vi "VM_ProjetoV5.1.vi"() -> ()   [LabVIEW 2016, in "Projeto_Modbus_Finalizado.lvlib"]
uses:
  Projeto_Modbus_Finalizado.lvlib
  <vilib>/userdefined/High Color/IMAQdx.ctl
  <vilib>/Analysis/baseanly.llb/Mean (DBL).vi
  <vilib>/lvdsc/process/Deploy Library.vi
  <vilib>/Utility/file.llb/Read Delimited Spreadsheet (DBL).vi
  <vilib>/Utility/file.llb/Write Delimited Spreadsheet (DBL).vi
  <vilib>/lvdsc/process/Undeploy Library.vi
  <vilib>/vision/driver/NI_Vision_Acquisition_Software.lvlib
  <resource>/objmgr/imaqdx.rc
  <vilib>/Analysis/NI_AALBase.lvlib
  <vilib>/lvdsc/NI_DSC.lvlib
panel:
  in  "Calibração\nRobô":path=path "C:/Users/rodrigorg1/Desktop/Projeto/calibracaoRobo.csv"
  in  "Calibração\nMesa":path=path "C:/Users/rodrigorg1/Desktop/Projeto/calibracaoMesa.csv"
  out "Error Out":errorcluster
  in  "Cut Limit":dbl=55.0 format="%#_13g"
  in  "Confirma":bool
  out "Status":string
  out "Câmera Robo":T1(plugin-control)
  out "Câmera Mesa":T1(plugin-control)
  in  "Começa jogada":bool
  in  "stop":bool
  in  "Source Câmera Robo":T2="S1156978"
  in  "Source Câmera Mesa":T2="cam0"
  out "Dobrao":bool
  out "Passa Vez":bool
  out "place pos Norm":dbl[](array[numeric])
  out "pick pos Norm":dbl[](array[numeric])
  out "place angle":dbl
  out "pick angle":dbl
  # "x 91\ny 176"
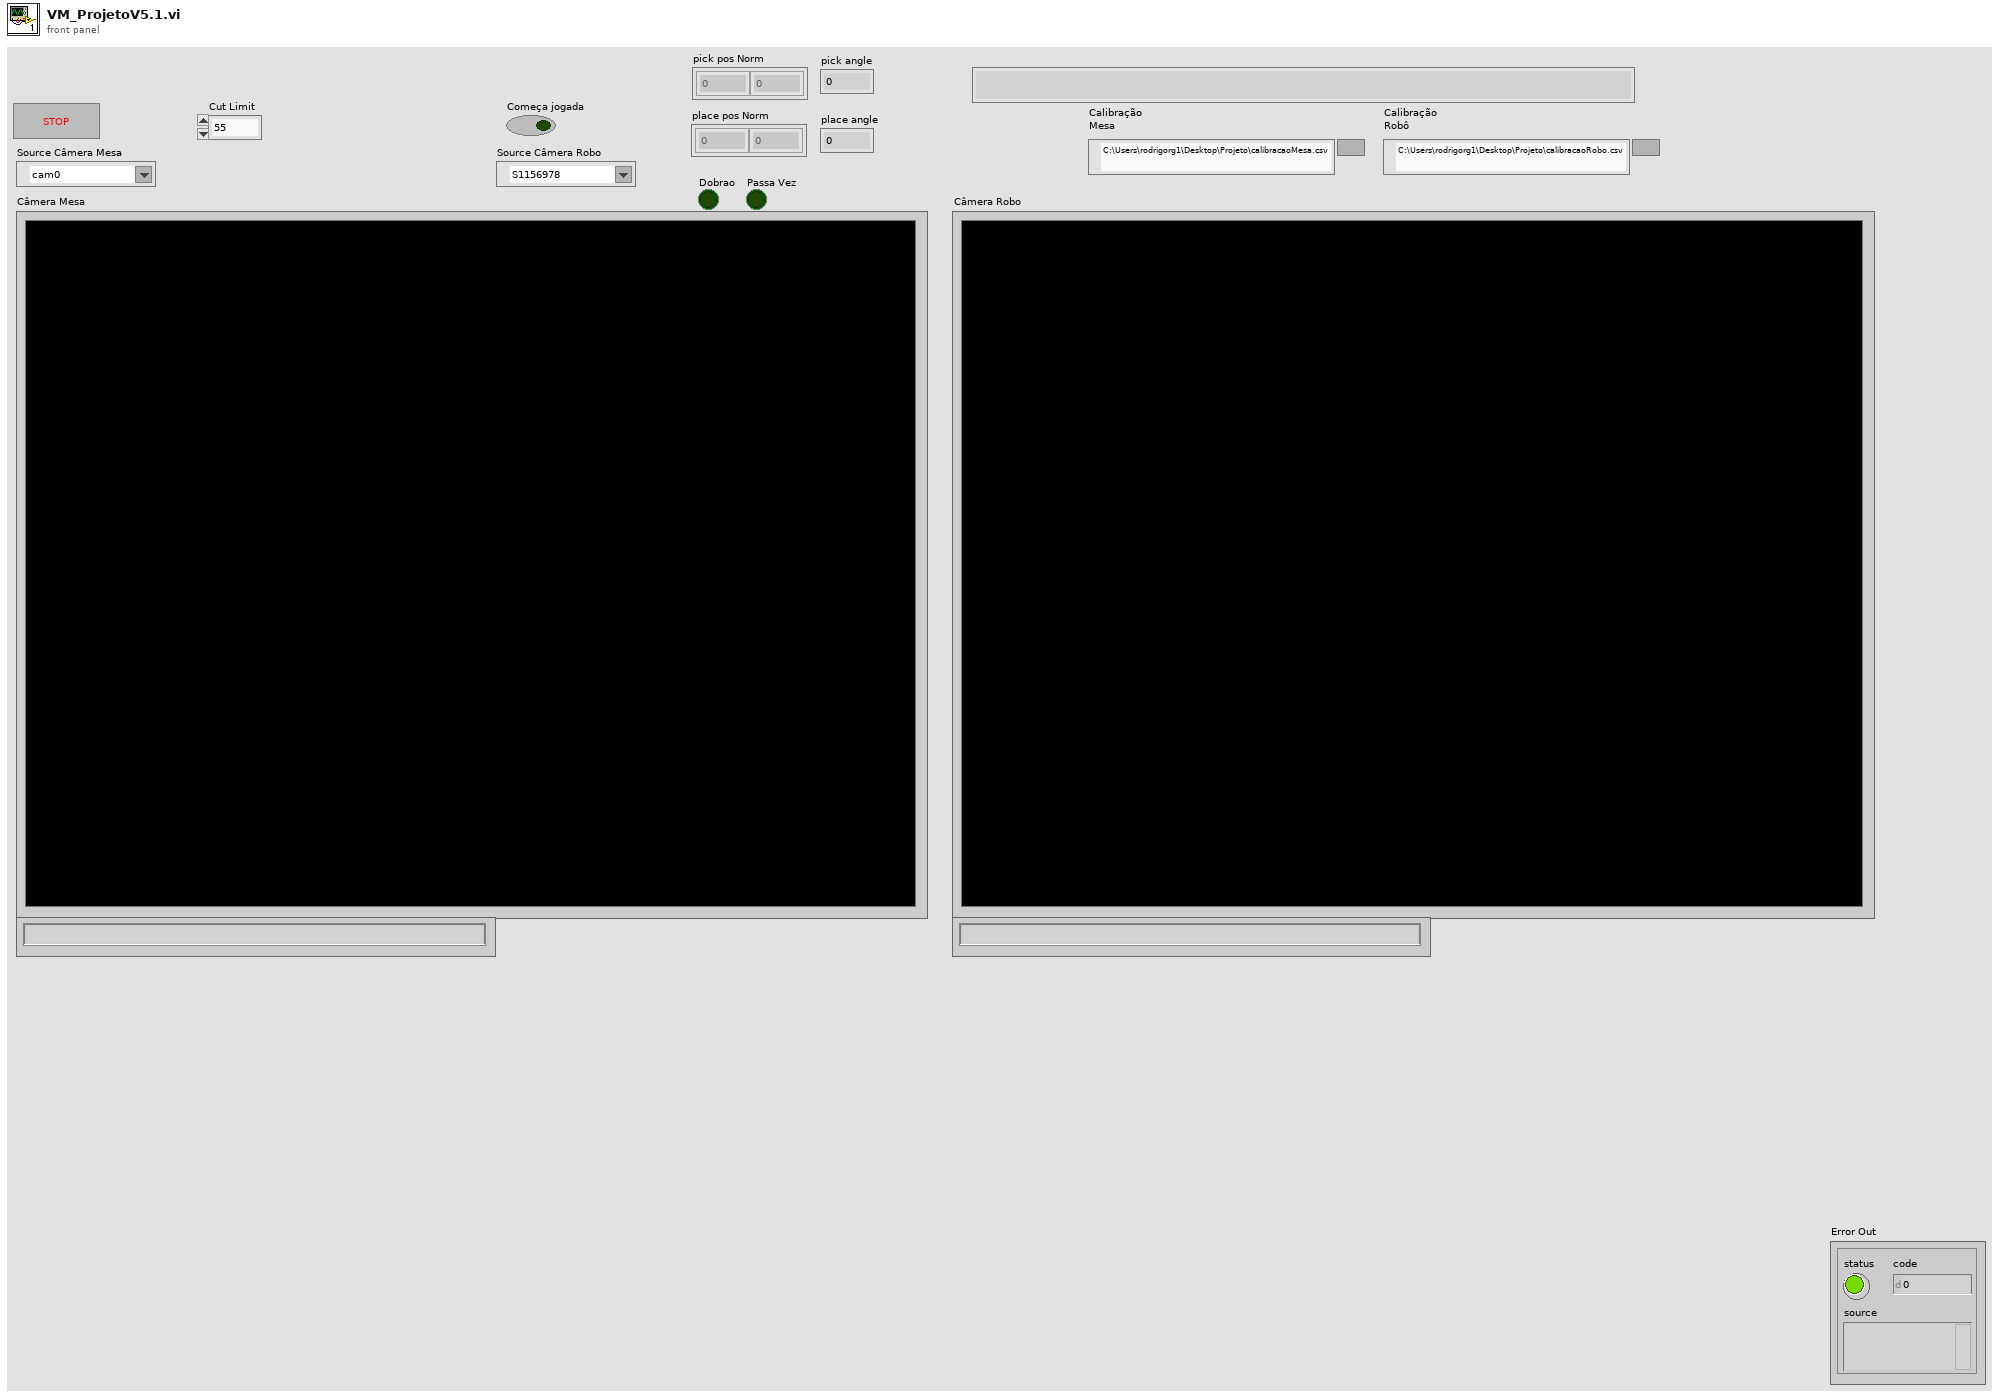
[diagram p1: front panel]
types:
  T1 = typedef "IMAQ Image.ctl" = refnum<image>
  T2 = typedef "IMAQdx.ctl" = refnum<k21>
  T3 = typedef "IMAQ Rectangle" = cluster{"Left":i32, "Top":i32, "Right":i32, "Bottom":i32, "Rotation":dbl}
  T4 = typedef "ROI Descriptor" = cluster{"Global Rectangle":i32[], "Contours":cluster{"ID":enum32{"External", "Internal"}, "Type":u32, "Coordinates":i32[]}[]}
  T5 = cluster{"Position":cluster{"x":sgl, "y":sgl}, "Angle":sgl, "Scale":sgl, "Score":sgl, "Bounding Box":cluster{"x":sgl, "y":sgl}[]}[]
  T6 = cluster{"Centro Peça":dbl[], "Centros Númeors":dbl[][], "Números":u8[], "ROI Números":T4[]}[]
  T7 = cluster{"Centro Peça":dbl[], "Centros Númeors":dbl[][], "Números":u8[], "ROI Números":T4[]}
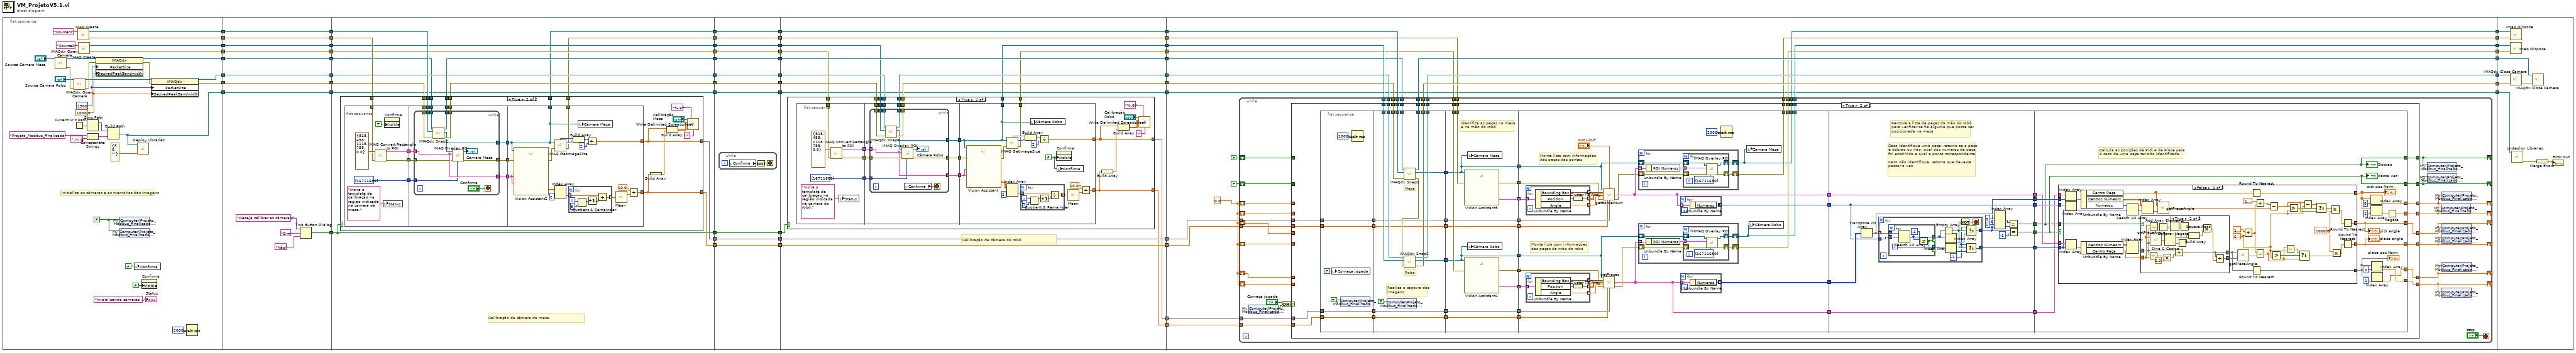
[diagram p0: block diagram]
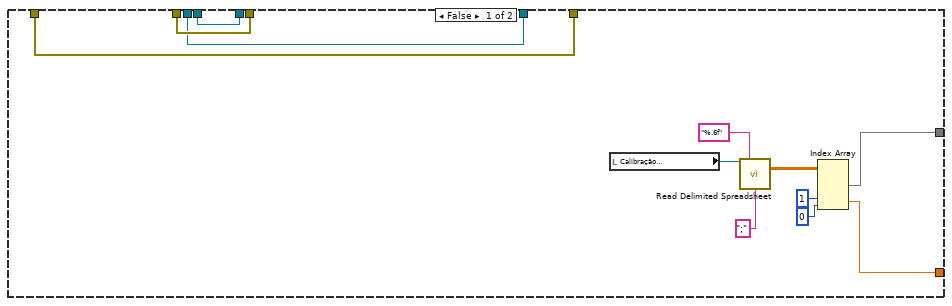
[diagram p2: hidden frame]
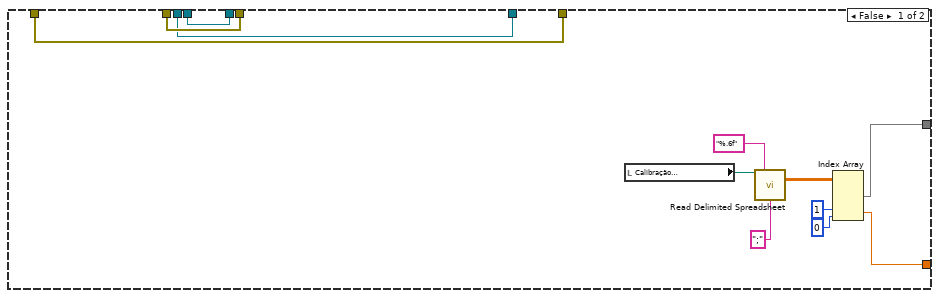
[diagram p3: hidden frame]
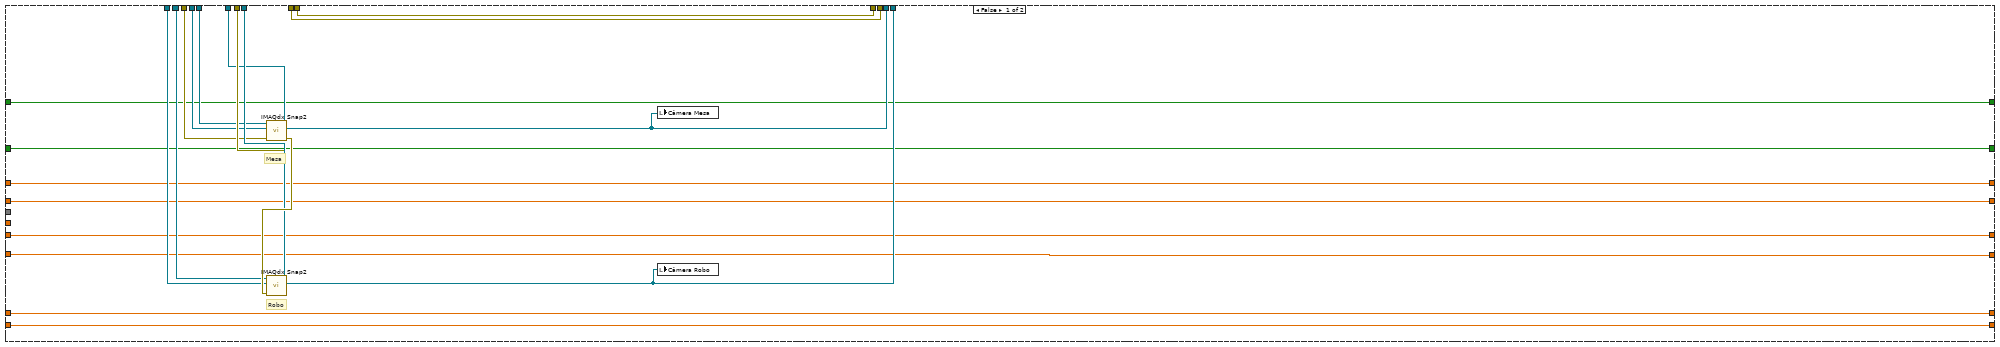
[diagram p4: hidden frame]
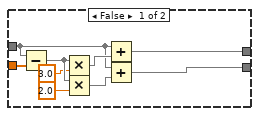
[diagram p5: hidden frame]
diagram:
  n1 = flat-sequence {
    tunnel: [w85] -> w17
    tunnel: [w84] -> w15
    tunnel: [w79] -> w13
    tunnel: [w83] -> w11
    tunnel: [w82] -> w9
    tunnel: [w78] -> w7
    tunnel: [w69] -> w5
    tunnel: [w61] -> w3
    tunnel: w17 -> [w101]
    tunnel: [w101] -> w16
    tunnel: w15 -> [w100]
    tunnel: [w100] -> w14
    tunnel: w13 -> [w99]
    tunnel: [w99] -> w12
    tunnel: w11 -> [w98]
    tunnel: [w98] -> w10
    tunnel: w9 -> [w97]
    tunnel: [w97] -> w8
    tunnel: w7 -> [w96]
    tunnel: [w96] -> w6
    tunnel: w5 -> [w95]
    tunnel: [w95] -> w4
    tunnel: w3 -> [w94]
    tunnel: [w94] -> w2
    tunnel: [w90] -> w1
    tunnel: w16 -> [w115]
    tunnel: w14 -> [w116]
    tunnel: w12 -> [w105]
    tunnel: w10 -> [w114]
    tunnel: w8 -> [w113]
    tunnel: w6 -> [w104]
    tunnel: [w109] -> w41
    tunnel: [w108] -> w39
    tunnel: [w114] -> w37
    tunnel: [w113] -> w35
    tunnel: [w112] -> w33
    tunnel: [w111] -> w31
    tunnel: w4 -> [w111]
    tunnel: [w110] -> w29
    tunnel: [w107] -> w27
    tunnel: [w106] -> w25
    tunnel: [w103] -> w20
    tunnel: w2 -> [w103]
    tunnel: [w102] -> w19
    tunnel: w1 -> [w102]
    tunnel: w41 -> [w213]
    tunnel: [w213] -> w40
    tunnel: w39 -> [w212]
    tunnel: [w212] -> w38
    tunnel: w37 -> [w211]
    tunnel: [w211] -> w36
    tunnel: w35 -> [w210]
    tunnel: [w210] -> w34
    tunnel: w33 -> [w209]
    tunnel: [w209] -> w32
    tunnel: w31 -> [w208]
    tunnel: [w208] -> w30
    tunnel: w29 -> [w207]
    tunnel: [w207] -> w28
    tunnel: w27 -> [w206]
    tunnel: [w206] -> w26
    tunnel: w25 -> [w205]
    tunnel: [w205] -> w24
    tunnel: [w204] -> w21
    tunnel: w20 -> [w204]
    tunnel: w19 -> [w203]
    tunnel: [w203] -> w18
    tunnel: w40 -> [w232]
    tunnel: [w232] -> w52
    tunnel: w38 -> [w231]
    tunnel: [w231] -> w51
    tunnel: w36 -> [w223]
    tunnel: [w222] -> w50
    tunnel: w34 -> [w221]
    tunnel: [w220] -> w49
    tunnel: w32 -> [w230]
    tunnel: [w230] -> w48
    tunnel: w30 -> [w225]
    tunnel: [w224] -> w47
    tunnel: w28 -> [w227]
    tunnel: [w226] -> w46
    tunnel: w26 -> [w229]
    tunnel: [w229] -> w45
    tunnel: w24 -> [w228]
    tunnel: [w228] -> w44
    tunnel: [w219] -> w43
    tunnel: [w218] -> w42
    tunnel: [w217] -> w22
    tunnel: w21 -> [w217]
    tunnel: w18 -> [w216]
    tunnel: [w337] -> w59
    tunnel: [w340] -> w58
    tunnel: [w334] -> w57
    tunnel: [w339] -> w56
    tunnel: [w338] -> w55
    tunnel: [w336] -> w54
    tunnel: [w335] -> w53
    tunnel: w52 -> [w333]
    tunnel: w51 -> [w332]
    tunnel: w50 -> [w331]
    tunnel: w49 -> [w330]
    tunnel: w48 -> [w329]
    tunnel: w47 -> [w328]
    tunnel: w46 -> [w327]
    tunnel: w45 -> [w325]
    tunnel: w44 -> [w326]
    tunnel: w43 -> [w323]
    tunnel: w42 -> [w324]
    tunnel: [w322] -> w23
    tunnel: w22 -> [w322]
    tunnel: w59 -> [w681]
    tunnel: w58 -> [w679]
    tunnel: w57 -> [w683]
    tunnel: w56 -> [w686]
    tunnel: w55 -> [w685]
    tunnel: w54 -> [w682]
    tunnel: w53 -> [w684]
    tunnel: w23 -> [w676]
    frame #0 {
      w60 = FALSE ("000021")
      w73 = 1000.0 ("DesiredPeakBandwidth")
      w74 = u32 1500 ("PacketSize")
      # "Inicializa as câmeras e as memórias das imagens"
      n2 = call <vilib>:"IMAQdx Open Camera.vi"("Session In"="Source Câmera Mesa") -> ("error out"=w77:errorcluster, "Session Out"=w80:T2)  [unwired: 9 in]
      n3 = Current VI's Path() -> (path=w62:path)
      n4 = call <vilib>:"IMAQdx Open Camera.vi"("error in"=w77, "Session In"="Source Câmera Robo") -> ("error out"=w76:errorcluster, "Session Out"=w81:T2)  [unwired: 8 in]
      n5 = call "IMAQ Create"("Image Name"="SourceM") -> ("New Image"=w85:T1, "error out"=w84:errorcluster)  [unwired: 4 in]
      n6 = call "IMAQ Create"("Image Name"="SourceR") -> ("New Image"=w83:T1, "error out"=w82:errorcluster)  [unwired: 4 in]
      n7 = Strip Path(path=w62) -> (stripped path=w63:path)  [unwired: 1 out]
      n8 = Concatenate Strings("Projeto_Modbus_Finalizado" ("library path"), ".lvlib" ("string")) -> (w66:string)
      n9 = property class="IMAQdx"(reference=w80, error in=w76, "PacketSize"=w74, "DesiredPeakBandwidth"=w73) -> (reference out=w79:T2, error out=w75:errorcluster)
      n10 = Build Path(base path=w63, name or relative path=w66) -> (appended path=w61:path)
      n11 = shared-variable "My Computer\\Projeto_Modbus_Finalizado.lvlib\\000021"(w60) -> ()  [unwired: 1 in, 1 out]
      n12 = shared-variable "My Computer\\Projeto_Modbus_Finalizado.lvlib\\000020"(w60) -> ()  [unwired: 1 in, 1 out]
      n13 = local write "Confirma"(FALSE ("Confirma")) -> ()
      n14 = call-poly <vilib>:"Deploy Libraries.vi"("error in (no error)"=errorcluster {"status"=FALSE, "code"=0, "source"=""}, "library path"=w61) -> ()  [unwired: 7 in, 1 out]
      n15 = property on="Confirma" class="Bool (strict)"("Visible"=FALSE) -> ()  [unwired: 2 in, 2 out]
      n16 = property class="IMAQdx"(reference=w81, error in=w75, "PacketSize"=w74, "DesiredPeakBandwidth"=w73) -> (reference out=w69:T2, error out=w78:errorcluster)
      n17 = Wait (ms)(milliseconds to wait=u32 2000) -> ()  [unwired: 1 out]
      "Status" <- "Inicializando câmeras ..." ("Status")
    }
    frame #1 {
      n18 = Two Button Dialog(message="Deseja calibrar as câmeras?", 1:"Não" ("F button name (\"Cancel\")"), 2:"Sim" ("T button name (\"OK\")")) -> (T button?=w90:bool)
    }
    frame #2 {
      # "Calibração da câmera da mesa"
      n19 = case shown="True" w102 {
        tunnel: w116 -> [w125 w143]
        tunnel: w115 -> [w126 w142]
        tunnel: [w127 w141] -> w112
        tunnel: [w128 w140] -> w110
        tunnel: [w126 w139] -> w109
        tunnel: [w125 w138] -> w108
        tunnel: [w118 w133] -> w107
        tunnel: [w117 w134] -> w106
        tunnel: w105 -> [w127 w137]
        tunnel: w104 -> [w128 w136]
        frame False {
          n20 = local read "Calibração\nMesa"() -> (w124:path)
          n21 = call-poly <vilib>:"Read Delimited Spreadsheet.vi"("file path (dialog if empty)"=w124, "format (%.3f)"="%.6f", "delimiter (\\t)"=";" ("delimiter (\\t)")) -> ("all rows"=w121:dbl[][])  [unwired: 7 in, 5 out]
          n22 = Index Array(array=w121, index (row) #2=1, index (col) #2=0) -> (element #1=w117:dbl[], element #2=w118:dbl)  [unwired: 2 in]
        }
        frame True {
          n23 = flat-sequence {
            tunnel: w143 -> [w154]
            tunnel: [w152] -> w149
            tunnel: [w151] -> w148
            tunnel: [u32[] [16711680] ("Colors (Green)")] -> w147
            tunnel: w137 -> [w167]
            tunnel: w136 -> [w166]
            tunnel: w142 -> [w165]
            tunnel: [w164] -> w141
            tunnel: [w163] -> w140
            tunnel: w149 -> [w162]
            tunnel: w148 -> [w161]
            tunnel: [w160] -> w146
            tunnel: [w159] -> w145
            tunnel: [w158] -> w144
            tunnel: w147 -> [w157]
            tunnel: w146 -> [w196]
            tunnel: w145 -> [w195]
            tunnel: [w187] -> w133
            tunnel: w144 -> [w180]
            tunnel: [w180] -> w139
            tunnel: [w182] -> w138
            tunnel: [w181] -> w134
            frame #0 {
              n24 = call "IMAQ Convert Rectangle to ROI"("error in (no error)"=w154, "Rectangle"=T3 {"Left"=818, "Top"=458, "Right"=1118, "Bottom"=758, "Rotation"=0.0}) -> ("error out"=w152:errorcluster, "ROI Descriptor"=w151:T4)  [unwired: 7 in]
              n25 = local write "Status"("Insira o template de calibração na região indicada na câmera da mesa." ("Status")) -> ()
              n26 = property on="Confirma" class="Bool (strict)"("Visible"=TRUE) -> ()  [unwired: 2 in, 2 out]
            }
            frame #1 {
              n27 = while {
                tunnel: w167 -> [w178]
                tunnel: w166 -> [w177]
                tunnel: w165 -> [w176]
                tunnel: [w175] -> w164
                tunnel: [w174] -> w163
                tunnel: w162 -> [w168]
                tunnel: w161 -> [w171]
                tunnel: [w173] -> w160
                tunnel: [w171] -> w159
                tunnel: [w169] -> w158
                tunnel: w157 -> [w170]
                stop <- "Confirma" stop-if-true
                n28 = call <vilib>:"IMAQdx Snap2.vi"("error in"=w177, "Image In"=w176, "Session In"=w178) -> ("error out"=w174:errorcluster, "Image Out"=w169:T1, "Session Out"=w175:T2)  [unwired: 6 in]
                n29 = call "IMAQ Overlay ROI"("Colors (Green)"=w170, "error in (no error)"=w168, "ROI Descriptor"=w171, "Image"=w169) -> ("error out"=w173:errorcluster, "Image Out"=→"Câmera Mesa":T1)  [unwired: 6 in]
              }
            }
            frame #2 {
              n30 = call "Vision Assistant2"("Image In"=w180, "ROI Descriptor (Adv. Straight Edge 1)"=w195, "ROI Descriptor (Copy of Adv. Straight Edge 1)"=w195, "error in"=w196) -> ("Caliper Results (Caliper 2)"=w194:sgl[][], "error out"=w188:errorcluster)  [unwired: 21 in, 1 out]
              n31 = call "IMAQ GetImageSize"("Image"=w180, "error in (no error)"=w188) -> ("Y Resolution"=w186:i32, "X Resolution"=w185:i32, "error out"=w182:errorcluster)  [unwired: 2 in]
              n32 = Index Array(array=w194, index (col)=2 ("disabled index (col)")) -> (element=w192:sgl[])  [unwired: 1 in]
              n33 = for {
                tunnel: w192 -> [w199] mode=indexing
                tunnel: [w197] -> w191 mode=indexing
                i -> [w202]
                n34 = Quotient & Remainder(x=w202, y=5) -> (x-y*floor(x/y)=w200:i32)  [unwired: 1 out]
                n35 = Increment(x=w200) -> (x+1=w198:i32)
                n36 = Divide(x=w199, y=w198) -> (x/y=w197:sgl)
              }
              n37 = Build Array(w185, w186) -> (w184:i32[])
              n38 = local write "Câmera Mesa"(w180) -> ()
              n39 = Divide(x=w184, y=2) -> (x/y=w181:dbl[])
              n40 = call-poly <vilib>:"Mean.vi"("X"=w191) -> ("mean"=w190:dbl)  [unwired: 1 out]
              n41 = Divide(x=10.0, y=w190) -> (x/y=w187:dbl)
            }
          }
          n42 = Build Array(w133) -> (w132:dbl[])
          n43 = Build Array(w134, w132) -> (w131:dbl[][])
          n44 = call-poly <vilib>:"Write Delimited Spreadsheet.vi"("file path (dialog if empty)"="Calibração\nMesa", "format (%.3f)"="%.6f", "2D data"=w131, "delimiter (\\t)"=";" ("delimiter (\\t)")) -> ()  [unwired: 10 in, 2 out]
        }
      }
    }
    frame #3 {
      n45 = while {
        stop <- w215 stop-if-true
        n46 = local read "Confirma"() -> (w214:bool)
        n47 = Not(x=w214) -> (.not. x?=w215:bool)
      }
    }
    frame #4 {
      # "Calibração da câmera do robô"
      n48 = case shown="True" w216 {
        tunnel: w227 -> [w243 w259]
        tunnel: [w243 w258] -> w226
        tunnel: w225 -> [w244 w257]
        tunnel: [w244 w256] -> w224
        tunnel: w223 -> [w242 w255]
        tunnel: [w242 w254] -> w222
        tunnel: w221 -> [w241 w253]
        tunnel: [w241 w252] -> w220
        tunnel: [w233 w246] -> w219
        tunnel: [w234 w245] -> w218
        frame False {
          n49 = local read "Calibração\nRobô"() -> (w235:path)
          n50 = call-poly <vilib>:"Read Delimited Spreadsheet.vi"("file path (dialog if empty)"=w235, "format (%.3f)"="%.6f", "delimiter (\\t)"=";" ("delimiter (\\t)")) -> ("all rows"=w238:dbl[][])  [unwired: 7 in, 5 out]
          n51 = Index Array(array=w238, index (row) #2=1, index (col) #2=0) -> (element #1=w234:dbl[], element #2=w233:dbl)  [unwired: 2 in]
        }
        frame True {
          n52 = flat-sequence {
            tunnel: w253 -> [w270]
            tunnel: [w269] -> w265
            tunnel: [w268] -> w264
            tunnel: [u32[] [16711680] ("Colors (Green)")] -> w263
            tunnel: w257 -> [w282]
            tunnel: w259 -> [w281]
            tunnel: w255 -> [w280]
            tunnel: [w279] -> w256
            tunnel: [w278] -> w258
            tunnel: w265 -> [w277]
            tunnel: w264 -> [w276]
            tunnel: [w275] -> w262
            tunnel: [w274] -> w261
            tunnel: [w273] -> w260
            tunnel: w263 -> [w272]
            tunnel: w262 -> [w312]
            tunnel: w261 -> [w311]
            tunnel: [w303] -> w246
            tunnel: w260 -> [w296]
            tunnel: [w296] -> w254
            tunnel: [w298] -> w252
            tunnel: [w297] -> w245
            frame #0 {
              n53 = call "IMAQ Convert Rectangle to ROI"("error in (no error)"=w270, "Rectangle"=T3 {"Left"=818, "Top"=458, "Right"=1118, "Bottom"=758, "Rotation"=0.0}) -> ("error out"=w269:errorcluster, "ROI Descriptor"=w268:T4)  [unwired: 7 in]
              n54 = local write "Status"("Insira o template de calibração na região indicada na câmera do robô." ("Status")) -> ()
            }
            frame #1 {
              n55 = while {
                tunnel: w282 -> [w294]
                tunnel: w281 -> [w293]
                tunnel: w280 -> [w292]
                tunnel: [w291] -> w279
                tunnel: [w290] -> w278
                tunnel: w277 -> [w289]
                tunnel: w276 -> [w287]
                tunnel: [w288] -> w275
                tunnel: [w287] -> w274
                tunnel: [w286] -> w273
                tunnel: w272 -> [w285]
                stop <- w283 stop-if-true
                n56 = call <vilib>:"IMAQdx Snap2.vi"("error in"=w293, "Image In"=w292, "Session In"=w294) -> ("error out"=w290:errorcluster, "Image Out"=w286:T1, "Session Out"=w291:T2)  [unwired: 6 in]
                n57 = call "IMAQ Overlay ROI"("Colors (Green)"=w285, "error in (no error)"=w289, "ROI Descriptor"=w287, "Image"=w286) -> ("error out"=w288:errorcluster, "Image Out"=→"Câmera Robo":T1)  [unwired: 6 in]
                n58 = local read "Confirma"() -> (w283:bool)
              }
            }
            frame #2 {
              w295 = FALSE ("Visible")
              n59 = call "Vision Assistant"("Image In"=w296, "ROI Descriptor (Adv. Straight Edge 1)"=w311, "ROI Descriptor (Copy of Adv. Straight Edge 1)"=w311, "error in"=w312) -> ("Caliper Results (Caliper 2)"=w310:sgl[][], "error out"=w304:errorcluster)  [unwired: 21 in, 1 out]
              n60 = call "IMAQ GetImageSize"("Image"=w296, "error in (no error)"=w304) -> ("Y Resolution"=w302:i32, "X Resolution"=w301:i32, "error out"=w298:errorcluster)  [unwired: 2 in]
              n61 = Index Array(array=w310, index (col)=2 ("disabled index (col)")) -> (element=w308:sgl[])  [unwired: 1 in]
              n62 = for {
                tunnel: w308 -> [w315] mode=indexing
                tunnel: [w313] -> w307 mode=indexing
                i -> [w318]
                n63 = Quotient & Remainder(x=w318, y=5) -> (x-y*floor(x/y)=w316:i32)  [unwired: 1 out]
                n64 = Increment(x=w316) -> (x+1=w314:i32)
                n65 = Divide(x=w315, y=w314) -> (x/y=w313:sgl)
              }
              n66 = Build Array(w301, w302) -> (w300:i32[])
              n67 = local write "Câmera Robo"(w296) -> ()
              n68 = Divide(x=w300, y=2) -> (x/y=w297:dbl[])
              n69 = property on="Confirma" class="Bool (strict)"("Visible"=w295) -> ()  [unwired: 2 in, 2 out]
              n70 = local write "Confirma"(w295) -> ()
              n71 = call-poly <vilib>:"Mean.vi"("X"=w307) -> ("mean"=w306:dbl)  [unwired: 1 out]
              n72 = Divide(x=10.0, y=w306) -> (x/y=w303:dbl)
            }
          }
          n73 = Build Array(w246) -> (w250:dbl[])
          n74 = Build Array(w245, w250) -> (w249:dbl[][])
          n75 = call-poly <vilib>:"Write Delimited Spreadsheet.vi"("file path (dialog if empty)"="Calibração\nRobô", "format (%.3f)"="%.6f", "2D data"=w249, "delimiter (\\t)"=";" ("delimiter (\\t)")) -> ()  [unwired: 10 in, 2 out]
        }
      }
    }
    frame #5 {
      w319 = 0.0 ("Numeric")
      n76 = while {
        tunnel: w329 -> [w378]
        tunnel: w333 -> [w377]
        tunnel: w331 -> [w376]
        tunnel: w328 -> [w375]
        tunnel: w327 -> [w374]
        tunnel: [w373] -> w340
        tunnel: [w372] -> w339
        tunnel: [w371] -> w338
        tunnel: w332 -> [w370]
        tunnel: w330 -> [w369]
        tunnel: [w368] -> w337
        tunnel: [w367] -> w334
        tunnel: [w365] -> w336
        tunnel: [w364] -> w335
        tunnel: w326 -> [w363]
        tunnel: w325 -> [w362]
        tunnel: w324 -> [w361]
        tunnel: w323 -> [w360]
        shift-right: [w356] -> _
        shift-left: FALSE -> [w347]
        shift-right: [w355] -> _
        shift-left: FALSE -> [w348]
        shift-right: [w354] -> _
        shift-left: w319 -> [w346]
        shift-right: [w353] -> _
        shift-left: w319 -> [w345]
        shift-right: [w352] -> _
        shift-left: w319 -> [w344]
        shift-right: [w351] -> _
        shift-left: w319 -> [w343]
        shift-right: [w350] -> _
        shift-left: w319 -> [w342]
        shift-right: [w349] -> _
        shift-left: w319 -> [w341]
        stop <- "stop" stop-if-true
        n77 = shared-variable "My Computer\\Projeto_Modbus_Finalizado.lvlib\\000022"() -> (w357:bool)  [unwired: 1 in, 1 out]
        n78 = Or(x="Começa jogada", y=w357) -> (x .or. y?=w359:bool)
        n79 = case shown="True" w359 {
          tunnel: w378 -> [w390 w456]
          tunnel: w377 -> [w389 w455]
          tunnel: w376 -> [w396 w454]
          tunnel: w375 -> [w395 w453]
          tunnel: w374 -> [w392 w452]
          tunnel: [w391 w451] -> w373
          tunnel: [w394 w450] -> w372
          tunnel: [w393 w449] -> w371
          tunnel: w370 -> [w399 w447]
          tunnel: w369 -> [w398 w445]
          tunnel: [w388 w413] -> w368
          tunnel: [w387 w414] -> w367
          tunnel: [w399 w411] -> w365
          tunnel: [w398 w412] -> w364
          tunnel: w363 -> [_ w400]
          tunnel: w362 -> [_ w427]
          tunnel: w361 -> [_ w402]
          tunnel: w360 -> [_ w401]
          tunnel: [w384 w410] -> w354
          tunnel: [w382 w409] -> w353
          tunnel: [w383 w408] -> w352
          tunnel: [w381 w407] -> w351
          tunnel: [w380 w406] -> w350
          tunnel: [w379 w405] -> w349
          tunnel: [w385 w404] -> w356
          tunnel: [w386 w403] -> w355
          tunnel: w348 -> [w386 _]
          tunnel: w347 -> [w385 _]
          tunnel: w346 -> [w384 _]
          tunnel: w345 -> [w382 _]
          tunnel: w344 -> [w383 _]
          tunnel: w343 -> [w381 _]
          tunnel: w342 -> [w380 _]
          tunnel: w341 -> [w379 _]
          frame False {
            # "Robo"
            # "Mesa"
            n80 = call <vilib>:"IMAQdx Snap2.vi"("error in"=w392, "Image In"=w389, "Session In"=w390) -> ("error out"=w397:errorcluster, "Image Out"=w388:T1, "Session Out"=w391:T2)  [unwired: 6 in]
            n81 = call <vilib>:"IMAQdx Snap2.vi"("error in"=w397, "Image In"=w396, "Session In"=w395) -> ("error out"=w393:errorcluster, "Image Out"=w387:T1, "Session Out"=w394:T2)  [unwired: 6 in]
            n82 = local write "Câmera Mesa"(w388) -> ()
            n83 = local write "Câmera Robo"(w387) -> ()
          }
          frame True {
            n84 = flat-sequence {
              tunnel: w401 -> [w460]
              tunnel: w402 -> [w461]
              tunnel: w427 -> [w462]
              tunnel: w400 -> [w463]
              tunnel: [w463] -> w418
              tunnel: [w462] -> w417
              tunnel: [w461] -> w416
              tunnel: [w460] -> w415
              tunnel: w456 -> [w479]
              tunnel: w455 -> [w478]
              tunnel: w454 -> [w477]
              tunnel: w453 -> [w476]
              tunnel: w452 -> [w470]
              tunnel: [w475] -> w451
              tunnel: [w474] -> w450
              tunnel: [w473] -> w449
              tunnel: [w472] -> w448
              tunnel: [w471] -> w446
              tunnel: [w468] -> w425
              tunnel: [w467] -> w423
              tunnel: [w466] -> w421
              tunnel: [w465] -> w420
              tunnel: w418 -> [w468]
              tunnel: w417 -> [w467]
              tunnel: w416 -> [w466]
              tunnel: w415 -> [w465]
              tunnel: w448 -> [w481]
              tunnel: w447 -> [w491]
              tunnel: w446 -> [w480]
              tunnel: w445 -> [w490]
              tunnel: [w489] -> w444
              tunnel: [w488] -> w443
              tunnel: [w480] -> w442
              tunnel: [w481] -> w441
              tunnel: [w487] -> w440
              tunnel: [w486] -> w439
              tunnel: [w485] -> w426
              tunnel: w425 -> [w485]
              tunnel: [w484] -> w424
              tunnel: w423 -> [w484]
              tunnel: [w483] -> w422
              tunnel: w421 -> [w483]
              tunnel: w420 -> [w482]
              tunnel: [w482] -> w419
              tunnel: w444 -> [w519]
              tunnel: w443 -> [w518]
              tunnel: w442 -> [w493]
              tunnel: w441 -> [w494]
              tunnel: w440 -> [w514]
              tunnel: w439 -> [w510]
              tunnel: [w509] -> w438
              tunnel: [w508] -> w437
              tunnel: [w502] -> w436
              tunnel: [w500] -> w435
              tunnel: w426 -> [w507]
              tunnel: w424 -> [w506]
              tunnel: w422 -> [w505]
              tunnel: w419 -> [w504]
              tunnel: [w495] -> w414
              tunnel: [w498] -> w412
              tunnel: [w496] -> w413
              tunnel: [w497] -> w411
              tunnel: w438 -> [w558]
              tunnel: w437 -> [w565]
              tunnel: w436 -> [w564]
              tunnel: w435 -> [w560]
              tunnel: [w564] -> w434
              tunnel: [w563] -> w433
              tunnel: [w562] -> w432
              tunnel: [w561] -> w431
              tunnel: [w560] -> w430
              tunnel: [w559] -> w429
              tunnel: [w558] -> w428
              tunnel: w434 -> [w605]
              tunnel: w433 -> [w595]
              tunnel: w432 -> [w596]
              tunnel: w431 -> [w608]
              tunnel: w430 -> [w604]
              tunnel: w429 -> [w607]
              tunnel: w428 -> [w606]
              tunnel: [w597] -> w410
              tunnel: [w589] -> w409
              tunnel: [w594] -> w408
              tunnel: [w593] -> w407
              tunnel: [w591] -> w406
              tunnel: [w592] -> w405
              tunnel: [w596] -> w404
              tunnel: [w595] -> w403
              frame #0 {
                n85 = local write "Começa jogada"(FALSE ("Começa jogada")) -> ()
                n86 = shared-variable "My Computer\\Projeto_Modbus_Finalizado.lvlib\\000021"(TRUE ("000021")) -> ()  [unwired: 1 in, 1 out]
                n87 = Wait (ms)(milliseconds to wait=u32 1000) -> ()  [unwired: 1 out]
              }
              frame #1 {
                # "Realiza a captura das\nimagens"
                # "Robo"
                # "Mesa"
                n88 = shared-variable "My Computer\\Projeto_Modbus_Finalizado.lvlib\\000021"(FALSE ("000021")) -> ()  [unwired: 1 in, 1 out]
                n89 = call <vilib>:"IMAQdx Snap2.vi"("error in"=w470, "Image In"=w478, "Session In"=w479) -> ("error out"=w469:errorcluster, "Image Out"=w472:T1, "Session Out"=w475:T2)  [unwired: 6 in]
                n90 = call <vilib>:"IMAQdx Snap2.vi"("error in"=w469, "Image In"=w477, "Session In"=w476) -> ("error out"=w473:errorcluster, "Image Out"=w471:T1, "Session Out"=w474:T2)  [unwired: 6 in]
              }
              frame #2 {
                # "Identifica as peças na mesa\ne na mão do robô"
                n91 = call "Vision Assistant3"("Image In"=w481, "error in"=w491) -> ("Matches (Pattern Matching 1)"=w488:T5, "error out"=w487:errorcluster)  [unwired: 23 in, 1 out]
                n92 = call "Vision Assistant4"("Image In"=w480, "error in"=w490) -> ("Matches (Pattern Matching 1)"=w489:T5, "error out"=w486:errorcluster)  [unwired: 23 in, 1 out]
                n93 = local write "Câmera Mesa"(w481) -> ()
                n94 = local write "Câmera Robo"(w480) -> ()
              }
              frame #3 {
                # "Monta lista com informações\ndas peças das pontas"
                # "Monta lista com informações\ndas peças da mão do robô"
                n95 = for {
                  tunnel: w518 -> [w552] mode=indexing
                  tunnel: [w550] -> w516 mode=indexing
                  tunnel: [w549] -> w517 mode=indexing
                  tunnel: [w548] -> w515 mode=indexing
                  n96 = Unbundle By Name(w552) -> ("Bounding Box"=w549:cluster{"x":sgl, "y":sgl}[], "Position"=w551:cluster{"x":sgl, "y":sgl}, "Angle"=w548:sgl)
                  n97 = Cluster To Array(cluster=w551) -> (array=w550:sgl[])
                }
                n98 = for {
                  tunnel: w519 -> [w557] mode=indexing
                  tunnel: [w555] -> w512 mode=indexing
                  tunnel: [w554] -> w513 mode=indexing
                  tunnel: [w553] -> w511 mode=indexing
                  n99 = Unbundle By Name(w557) -> ("Bounding Box"=w554:cluster{"x":sgl, "y":sgl}[], "Position"=w556:cluster{"x":sgl, "y":sgl}, "Angle"=w553:sgl)
                  n100 = Cluster To Array(cluster=w556) -> (array=w555:sgl[])
                }
                n101 = call "getBorderNum.vi"("Refnum in"=w494, "Cut Limit"="Cut Limit", "Bounding Box"=w517, "Position"=w516, "Angle"=w515, "error in (no error)"=w514, "Step"=w506, "Origin Pixel"=w507) -> ("Data Pieces"=w502:T6, "error out"=w501:errorcluster)  [unwired: 5 in, 1 out]
                n102 = call "getPieces.vi"("Refnum in"=w493, "Bounding Box"=w513, "Position"=w512, "Angle"=w511, "error in (no error)"=w510, "Step"=w504, "Origin Pixel"=w505) -> ("Data Pieces"=w500:T6, "error out"=w499:errorcluster)  [unwired: 6 in, 1 out]
                n103 = for {
                  tunnel: w502 -> [w537] mode=indexing
                  shift-right: [w534] -> w496
                  shift-left: w494 -> [w535]
                  shift-right: [w532] -> w497
                  shift-left: w501 -> [w533]
                  n104 = Unbundle By Name(w537) -> ("ROI Números"=w536:T4[])
                  n105 = for {
                    tunnel: w536 -> [w543] mode=indexing
                    shift-right: [w541] -> w534
                    shift-left: w535 -> [w542]
                    shift-right: [w539] -> w532
                    shift-left: w533 -> [w540]
                    n106 = call "IMAQ Overlay ROI"("Colors (Green)"=u32[] [16711680], "error in (no error)"=w540, "ROI Descriptor"=w543, "Image"=w542) -> ("error out"=w539:errorcluster, "Image Out"=w541:T1)  [unwired: 6 in]
                  }
                }
                n107 = for {
                  tunnel: w500 -> [w525] mode=indexing
                  shift-right: [w522] -> w495
                  shift-left: w493 -> [w523]
                  shift-right: [w520] -> w498
                  shift-left: w499 -> [w521]
                  n108 = Unbundle By Name(w525) -> ("ROI Números"=w524:T4[])
                  n109 = for {
                    tunnel: w524 -> [w531] mode=indexing
                    shift-right: [w529] -> w522
                    shift-left: w523 -> [w530]
                    shift-right: [w527] -> w520
                    shift-left: w521 -> [w528]
                    n110 = call "IMAQ Overlay ROI"("Colors (Green)"=u32[] [16711680], "error in (no error)"=w528, "ROI Descriptor"=w531, "Image"=w530) -> ("error out"=w527:errorcluster, "Image Out"=w529:T1)  [unwired: 6 in]
                  }
                }
                n111 = for {
                  tunnel: w502 -> [w547] mode=indexing
                  tunnel: [w546] -> w509 mode=concatenating
                  n112 = Unbundle By Name(w547) -> ("Números"=w546:u8[])
                }
                n113 = for {
                  tunnel: w500 -> [w545] mode=indexing
                  tunnel: [w544] -> w508 mode=indexing
                  n114 = Unbundle By Name(w545) -> ("Números"=w544:u8[])
                }
                n115 = Wait (ms)(milliseconds to wait=u32 2000) -> ()  [unwired: 1 out]
                n116 = local write "Câmera Mesa"(w496) -> ()
                n117 = local write "Câmera Robo"(w495) -> ()
              }
              frame #4 {
                # "Caso identifique uma peça, retorna se a peça\né dobrão ou não, qual dos números da peça\nfoi escolhida e qual a ponta correspondente.\n\nCaso não identifique, retorna que deve-se\npassar a vez."
                # "Percorre a lista de peças da mão do robô\npara verificar se há alguma que possa ser\nposicionada na mesa"
                n118 = Transpose 2D Array(2D array=w565) -> (transposed array=w567:u8[][])
                n119 = for {
                  tunnel: w567 -> [w582] mode=indexing
                  tunnel: w558 -> [w581]
                  tunnel: [w573] -> w561
                  tunnel: [w572] -> w559
                  stop <- w577 stop-if-true
                  w574 = -1 ("t")
                  n120 = for {
                    tunnel: w582 -> [w588]
                    tunnel: w581 -> [w587] mode=indexing
                    tunnel: [w585] -> w579 mode=indexing if=w583
                    tunnel: [w584] -> w578 mode=indexing if=w583
                    i -> [w584]
                    n121 = Search 1D Array(1D array=w588, element=w587) -> (index of element=w585:i32)  [unwired: 1 in]
                    n122 = Not Equal?(x=w585, y=-1) -> (x != y?=w583:bool)
                  }
                  n123 = Empty Array?(array=w579) -> (empty?=w575:bool)
                  n124 = Index Array(array=w579) -> (element=w580:i32)  [unwired: 1 in]
                  n125 = Index Array(array=w578) -> (element=w576:i32)  [unwired: 1 in]
                  n126 = Not(x=w575) -> (.not. x?=w577:bool)
                  n127 = Select(t=w574, s=w575, f=w580) -> (s? t:f=w572:i32)
                  n128 = Select(t=w574, s=w575, f=w576) -> (s? t:f=w573:i32)
                }
                n129 = Index Array(array=w567, index (row) #1=0 ("disabled index (row)"), index (col) #1=w559, index (row) #2=1 ("disabled index (row)"), index (col) #2=w559) -> (element #1=w571:u8, element #2=w570:u8)
                n130 = Equal?(x=w571, y=w570) -> (x = y?=w563:bool)
                n131 = Equal?(x=w559, y=-1) -> (x = y?=w562:bool)
              }
              frame #5 {
                # "Calcula as posições de Pick e de Place para\no caso de uma peça ter sido identificada."
                n132 = case shown="False" w596 {
                  tunnel: w604 -> [w645 _]
                  tunnel: w607 -> [w644 _]
                  tunnel: w608 -> [w641 _]
                  tunnel: w605 -> [w643 _]
                  tunnel: w606 -> [w633 _]
                  tunnel: w595 -> [w638 _]
                  tunnel: [w631 _] -> w602
                  tunnel: [w630 _] -> w598
                  tunnel: [w626 _] -> w593
                  tunnel: [w627 _] -> w594
                  frame False {
                    w614 = 6.283185307179586
                    w632 = 1000.0
                    n133 = Index Array(array=w645, index=w644) -> (element=w646:T7)
                    n134 = Index Array(array=w633, index=w641) -> (element=w640:u8)
                    n135 = Index Array(array=w643, index=w641) -> (element=w642:T7)
                    n136 = Unbundle By Name(w646) -> ("Centro Peça"=w628:dbl[], "Centros Númeors"=w648:dbl[][], "Números"=w647:u8[])
                    n137 = Unbundle By Name(w642) -> ("Centros Númeors"=w635:dbl[][], "Centro Peça"=w634:dbl[])
                    n138 = Search 1D Array(1D array=w647, element=w640) -> (index of element=w649:i32)  [unwired: 1 in]
                    n139 = Index Array(array=w635) -> (element=w637:dbl[])  [unwired: 2 in]
                    n140 = case shown="True" w638 {
                      tunnel: w637 -> [w653 w668]
                      tunnel: w634 -> [w657 w669]
                      tunnel: [w651 w661] -> w636
                      tunnel: [w650 w660] -> w629
                      frame False {
                        n141 = Subtract(x=w653, y=w657) -> (x-y=w656:dbl[])
                        n142 = Multiply(x=w656, y=3.0) -> (x*y=w658:dbl[])
                        n143 = Multiply(x=w656, y=2.0) -> (x*y=w652:dbl[])
                        n144 = Add(x=w653, y=w658) -> (x+y=w650:dbl[])
                        n145 = Add(x=w653, y=w652) -> (x+y=w651:dbl[])
                      }
                      frame True {
                        n146 = Subtract(x=w668, y=w669) -> (x-y=w675:dbl[])
                        n147 = Subtract(x=w669, y=w668) -> (x-y=w672:dbl[])
                        n148 = call "getPieceAngle.vi"("Center Num"=w668, "Center Piece"=w669) -> ("Angle"=w667:dbl)
                        n149 = Square(x=w672) -> (x^2=w671:dbl[])
                        n150 = Multiply(x=w675, y=2.0) -> (x*y=w673:dbl[])
                        n151 = Sine & Cosine(0:w667) -> (1:w665:dbl, 2:w666:dbl)
                        n152 = Add Array Elements(numeric array=w671) -> (sum=w670:dbl)
                        n153 = Add(x=w668, y=w673) -> (x+y=w660:dbl[])
                        n154 = Negate(x=w666) -> (-x=w664:dbl)
                        n155 = Square Root(x=w670) -> (sqrt(x)=w662:dbl)
                        n156 = Build Array(w664, w665) -> (w663:dbl[])
                        n157 = Multiply(x=w662, y=w663) -> (x*y=w659:dbl[])
                        n158 = Add(x=w660, y=w659) -> (x+y=w661:dbl[])
                      }
                    }
                    n159 = Index Array(array=w648, index (row)=w649) -> (element=w639:dbl[])  [unwired: 1 in]
                    n160 = call "getPieceAngle.vi"("Center Num"=w639, "Center Piece"=w628) -> ("Angle"=w622:dbl)
                    n161 = call "getPieceAngle.vi"("Center Num"=w636, "Center Piece"=w629) -> ("Angle"=w623:dbl)
                    n162 = Add(x=1.5707963267948966, y=w614) -> (x+y=w611:dbl)
                    n163 = Round To Nearest(number=w628) -> (nearest integer value=w631:dbl[])
                    n164 = Round To Nearest(number=w629) -> (nearest integer value=w630:dbl[])
                    n165 = Add(x=1.5707963267948966, y=w611) -> (x+y=w610:dbl)
                    n166 = Subtract(x=w611, y=w623) -> (x-y=w615:dbl)
                    n167 = Subtract(x=w610, y=w622) -> (x-y=w618:dbl)
                    n168 = Greater?(x=w615, y=w614) -> (0:w620:bool)
                    n169 = Subtract(x=w615, y=w614) -> (x-y=w616:dbl)
                    n170 = Greater?(x=w618, y=w614) -> (0:w619:bool)
                    n171 = Select(t=w616, s=w620, f=w615) -> (s? t:f=w612:dbl)
                    n172 = Subtract(x=w618, y=w614) -> (x-y=w617:dbl)
                    n173 = Select(t=w617, s=w619, f=w618) -> (s? t:f=w613:dbl)
                    n174 = Multiply(x=w613, y=w632) -> (x*y=w625:dbl)
                    n175 = Multiply(x=w632, y=w612) -> (x*y=w624:dbl)
                    n176 = Round To Nearest(number=w625) -> (nearest integer value=w627:dbl)
                    n177 = Round To Nearest(number=w624) -> (nearest integer value=w626:dbl)
                  }
                  frame True {
                  }
                }
                "pick angle" <- w594
                "pick pos Norm" <- w602
                "place angle" <- w593
                "place pos Norm" <- w598
                n178 = Index Array(array=w602, index=0) -> (element=w597:dbl)
                n179 = Index Array(array=w602, index=1) -> (element=w590:dbl)
                n180 = Index Array(array=w598, index=0) -> (element=w592:dbl)
                n181 = Index Array(array=w598, index=1) -> (element=w591:dbl)
                n182 = Negate(x=w590) -> (-x=w589:dbl)
                "Passa Vez" <- w596
                "Dobrao" <- w595
              }
            }
          }
        }
        n183 = shared-variable "My Computer\\Projeto_Modbus_Finalizado.lvlib\\000018"(w355) -> ()  [unwired: 1 in, 1 out]
        n184 = shared-variable "My Computer\\Projeto_Modbus_Finalizado.lvlib\\000019"(w356) -> ()  [unwired: 1 in, 1 out]
        n185 = shared-variable "My Computer\\Projeto_Modbus_Finalizado.lvlib\\400130"(w353) -> ()  [unwired: 1 in, 1 out]
        n186 = shared-variable "My Computer\\Projeto_Modbus_Finalizado.lvlib\\400129"(w354) -> ()  [unwired: 1 in, 1 out]
        n187 = shared-variable "My Computer\\Projeto_Modbus_Finalizado.lvlib\\400133"(w352) -> ()  [unwired: 1 in, 1 out]
        n188 = shared-variable "My Computer\\Projeto_Modbus_Finalizado.lvlib\\400134"(w351) -> ()  [unwired: 1 in, 1 out]
        n189 = shared-variable "My Computer\\Projeto_Modbus_Finalizado.lvlib\\400131"(w350) -> ()  [unwired: 1 in, 1 out]
        n190 = shared-variable "My Computer\\Projeto_Modbus_Finalizado.lvlib\\400132"(w349) -> ()  [unwired: 1 in, 1 out]
      }
    }
    frame #6 {
      n191 = call "Imaq Dispose"("Image"=w681, "error in (no error)"=w682) -> ()  [unwired: 4 in, 1 out]
      n192 = call "Imaq Dispose"("Image"=w683, "error in (no error)"=w684) -> ()  [unwired: 4 in, 1 out]
      n193 = call <vilib>:"IMAQdx Close Camera.vi"("error in"=w685, "Session In"=w686) -> ("error out"=w680:errorcluster)  [unwired: 9 in]
      n194 = call-poly <vilib>:"Undeploy Libraries.vi"("library path"=w676) -> ("error out"=w678:errorcluster)  [unwired: 8 in]
      n195 = call <vilib>:"IMAQdx Close Camera.vi"("error in"=w680, "Session In"=w679) -> ()  [unwired: 9 in, 1 out]
      n196 = Merge Errors(w678) -> (→"Error Out":errorcluster)
    }
  }
